vi "Transform Paths to Net Use Paths.vi"(0 "Paths to be Mapped":path[](array[path]), 5 "Login Credentials":T1, 11 "error in":errorcluster) -> (4 "Transformed Paths":path[](array[path]), 6 "Mapped Drive Letters":string[](array[string]), 15 "error out":errorcluster)   [LabVIEW 2017, in "G3_Build Process File Utilities.lvlib"]
doc: "Transformas the array of input paths into paths that use a network mapped drive letter. If an input uses a network path, the first available drive leter is used to map to the share. One drive letter will be used per unique share in the array of paths. All mapped drive letters are retunred from this vi."
uses:
  G3_Build Process File Utilities.lvlib
  Net Use Login Credentials.ctl
  <userlib>/_OpenG.lib/array/array.llb/Filter 1D Array (String)__ogtk.vi
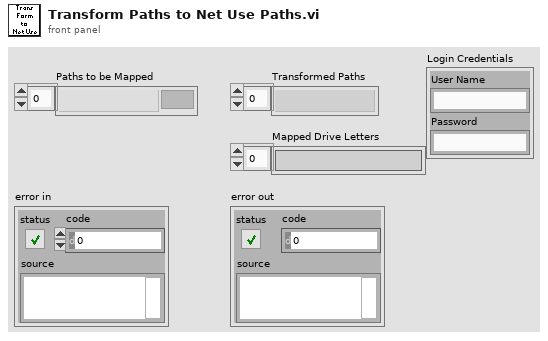
[diagram p1: front panel]
types:
  T1 = typedef "G3_Build Process File Utilities.lvlib/Net Use Login Credentials.ctl" = cluster{"User Name":string, "Password":string}
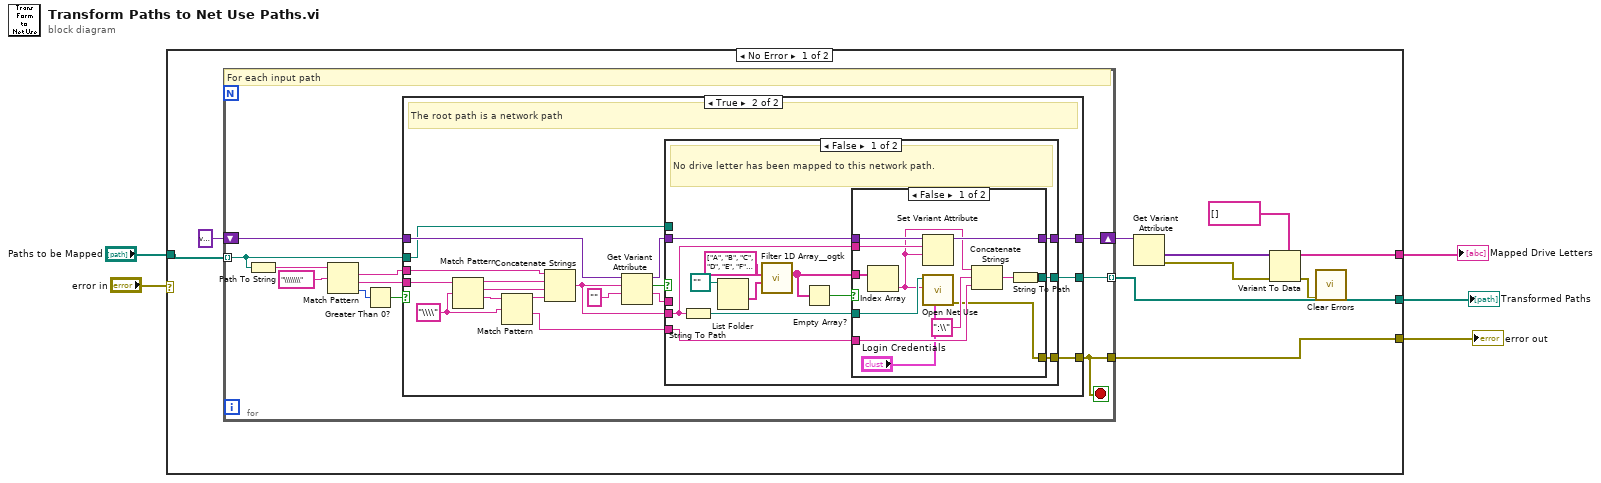
[diagram p0: block diagram]
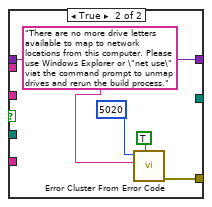
[diagram p3: hidden frame]
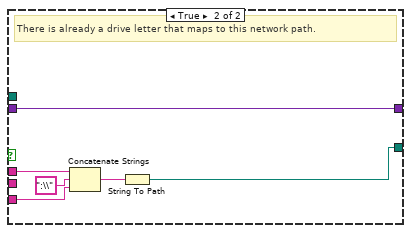
[diagram p4: hidden frame]
diagram:
  n1 = case shown="No Error" "error in" {
    selector: "error in" -> [_ w82]
    tunnel: [w15 _] -> w5
    tunnel: "Paths to be Mapped" -> [w14 _]
    tunnel: [w12 _] -> w3
    tunnel: [w8 w82] -> w2
    frame No Error {
      n2 = for {
        tunnel: w14 -> [w18] mode=indexing
        shift-right: [w19] -> w13
        shift-left: variant -> [w26]
        tunnel: [w17] -> w15 mode=indexing
        tunnel: [w16] -> w8
        stop <- w16 stop-if-true
        # "For each input path"
        n3 = Path To String(path=w18) -> (string=w20:string)
        n4 = Match Pattern(string=w20, regular expression="\\\\\\\\") -> (match substring=w21:string, after substring=w22:string, offset past match=w24:i32)  [unwired: 1 in, 1 out]
        n5 = Greater Than 0?(x=w24) -> (x > 0?=w23:bool)
        n6 = case shown="True" w23 {
          tunnel: w26 -> [w28 w46]
          tunnel: w22 -> [_ w45]
          tunnel: w21 -> [_ w44]
          tunnel: [w28 w38] -> w19
          tunnel: w18 -> [w27 w41]
          tunnel: [w27 w35] -> w17
          tunnel: [_ w29] -> w16
          frame False {
            # "This is not a network path"
          }
          frame True {
            w33 = "\\\\" ("regular expression")
            # "The root path is a network path"
            n7 = Match Pattern(string=w45, regular expression=w33) -> (before substring=w43:string, match substring=w32:string, after substring=w34:string)  [unwired: 1 in, 1 out]
            n8 = Match Pattern(string=w34, regular expression=w33) -> (before substring=w31:string, after substring=w30:string)  [unwired: 1 in, 2 out]
            n9 = Concatenate Strings(w44, w43, w32, w31) -> (w37:string)
            n10 = Get Variant Attribute(Variant=w46, name=w37, default value (empty Variant)="") -> (duplicate Variant=w39:variant, found=w42:bool, value=w40:string)  [unwired: 1 in, 1 out]
            n11 = case shown="False" w42 {
              tunnel: w41 -> [_ _]
              tunnel: w40 -> [_ w80]
              tunnel: w39 -> [w58 w81]
              tunnel: [w57 w81] -> w38
              tunnel: w37 -> [w50 _]
              tunnel: w30 -> [w53 w78]
              tunnel: [w52 w76] -> w35
              tunnel: [w47 _] -> w29
              frame False {
                # "No drive letter has been mapped to this network path."
                n12 = String To Path(string=w50) -> (path=w51:path)
                n13 = List Folder(path=path "") -> (folder names=w55:string[])  [unwired: 3 in, 3 out]
                n14 = call-poly <userlib>:"Filter 1D Array__ogtk.vi"("items to filter"=w55, "array"=string[] ["A", "B", "C", "D", "E", "F", "G", "H", "I", "J", "K", "L", "M", "N", "O", "P", "Q", "R", "S", "T", "U", "V", "W", "X", "Y", "Z"] ("Array")) -> ("filtered array"=w49:string[])  [unwired: 4 in, 1 out]
                n15 = Empty Array?(array=w49) -> (empty?=w48:bool)
                n16 = case shown="False" w48 {
                  tunnel: w58 -> [w70 w75]
                  tunnel: [w69 w75] -> w57
                  tunnel: w53 -> [w67 _]
                  tunnel: [w66 _] -> w52
                  tunnel: w51 -> [w64 _]
                  tunnel: w50 -> [w63 _]
                  tunnel: w49 -> [w61 _]
                  tunnel: [w60 w74] -> w47
                  frame False {
                    n17 = Index Array(array=w61) -> (element=w62:string)  [unwired: 1 in]
                    n18 = Set Variant Attribute(Variant=w70, name=w63, value=w62) -> (Variant out=w69:variant)  [unwired: 1 in, 2 out]
                    n19 = call "Open Net Use.vi"("Login Credentials"="Login Credentials", "Drive Letter (Y)"=w62, "Net Use Path"=w64) -> ("error IO"=w60:errorcluster)  [unwired: 6 in, 2 out]
                    n20 = Concatenate Strings(w62, ":\\" ("string"), w67) -> (w65:string)
                    n21 = String To Path(string=w65) -> (path=w66:path)
                  }
                  frame True {
                    n22 = call <vilib>:"Error Cluster From Error Code.vi"("show call chain? (False)"=TRUE, "error message (\"\")"="There are no more drive letters available to map to network locations from this computer. Please use Windows Explorer or \"net use\" viat the command prompt to unmap drives and rerun the build process." ("error message (\"\")"), "error code (0)"=5020) -> ("error out"=w74:errorcluster)  [unwired: 6 in]
                  }
                }
              }
              frame True {
                # "There is already a drive letter that maps to this network path."
                n23 = Concatenate Strings(w80, ":\\" ("string"), w78) -> (w77:string)
                n24 = String To Path(string=w77) -> (path=w76:path)
              }
            }
          }
        }
      }
      n25 = Get Variant Attribute(Variant=w13) -> (values=w11:variant[], error out=w7:errorcluster)  [unwired: 3 in, 2 out]
      n26 = Variant To Data(error in=w7, type=string[] [], Variant=w11) -> (data=w12:string[], error out=w6:errorcluster)
      n27 = call <vilib>:"Clear Errors.vi"("error in (no error)"=w6) -> ()  [unwired: 5 in, 2 out]
    }
    frame Error {
    }
  }
  "Transformed Paths" <- w5
  "Mapped Drive Letters" <- w3
  "error out" <- w2
